vi "Get Search Replace Strings.vi"(10 "New Name":string="test", 11 "GUID":string="test") -> (2 "Replacement Strings":string[](array[string]), 3 "Search Strings":string[](array[string]))   [LabVIEW 2020, in "ADAS_IO_Template_MDO.lvclass"]
uses:
  ADAS_IO_Template_MDO.lvclass
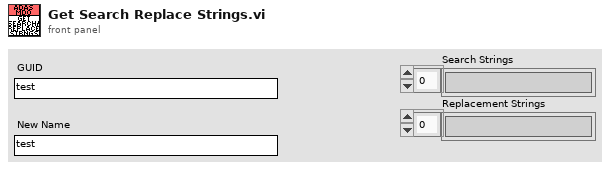
[diagram p1: front panel]
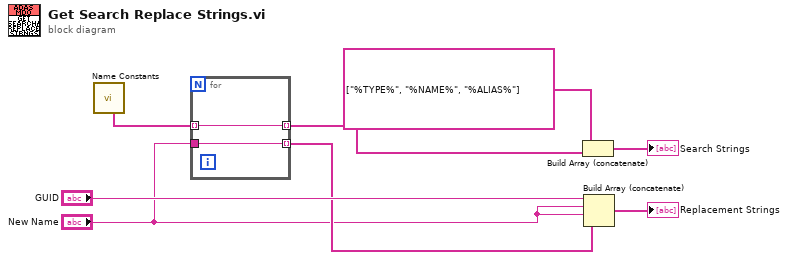
[diagram p0: block diagram]
diagram:
  n1 = call "Name Constants.vi"() -> ("Strings to Replace w Name"=w5:string[])  [unwired: 9 in, 2 out]
  n2 = for {
    tunnel: w5 -> [w9] mode=indexing
    tunnel: "New Name" -> [w10]
    tunnel: [w10] -> w4 mode=indexing
    tunnel: [w9] -> w3 mode=indexing
  }
  n3 = Build Array (concatenate)(string[] ["%TYPE%", "%NAME%", "%ALIAS%"], w3) -> (→"Search Strings":string[])
  n4 = Build Array (concatenate)("GUID", "New Name", "New Name", w4) -> (→"Replacement Strings":string[])
